vi "UI_Get_Application_Infos.vi"(8 "error in (no error)":errorcluster, 11 "Variant":variant) -> (0 "error out":errorcluster caption="sortie d'erreur", 3 "Variant Output":variant)   [LabVIEW 2018]
uses:
  controls/EXPERT_Inputs.ctl
  controls/DIGIT_5122_Inputs.ctl
  <instrlib>/niScope/Controls/niScope trigger source.ctl
  controls/HSDIO_6541_Inputs.ctl
  <instrlib>/niHSDIO/niHSDIO.llb/niHSDIO_ctl Trigger Source Values (Ring).ctl
  controls/SOFTWARE_Inputs.ctl
  controls/AO_6711_Inputs.ctl
  controls/AWG_5421_Inputs.ctl
  <instrlib>/niFgen/niFgen.llb/niFgen_ctl Trigger Source Values (Ring).ctl
  controls/XML_Inputs.ctl
  controls/EXPERT_Path_Selector.ctl
panel:
  in  "EXPERT Inputs":T1={"DIGIT 5122 Inputs"={"Sample Rate"=9.0, "Resource Name"="Digitizer", "Channel Name"="0", "Trigger Source"="VAL_EXTERNAL", "Vertical Range"=10.0, "Trigger Level"=3.0}, "HSDIO 6541 Inputs"={"Resource Name"="SequencerHSDIO", "Clock Rate"=1000000.0, "Trigger Source"="PFI0"}, "SOFTWARE Inputs"={"Application Directory"=path "D:/S.O.F.T.S/LABVIEW/PIL", "Software Version"="1.0.0", "Data Path"=path "D:/PIRENEA/DATA", "XML Path"=path "D:/PIRENEA/DATA", "XML File Filter"="*.xml", "XML Saved Path"=path "D:/PIRENEA/DATA", "Excit Scripts Path"=path "D:/PIRENEA/EXCIT_SCRIPTS", "Excit Scripts File Filter"="*.txt", "Excit Waveforms Path"=path "D:/PIRENEA/EXCIT_WFMS", "Excit Waveforms File Filter"="*.bin", "Timing Scripts Path"=path "D:/PIRENEA/SEQUENCE_SCRIPTS", "Timing Scripts File Filter"="*.txt", "Timing Waveforms Path"=path "D:/PIRENEA/SEQUENCE_WFMS", "Timing Waveforms File Filter"="*.bin", "Trapping Waveforms Path"=path "D:/PIRENEA/TRAPPING_WFMS", "Trapping Waveforms File Filter"="*.bin"}, "AO 6711 Inputs"={"Physical Channels"="AnalogOutput/ao0:3", "Min Voltage"=-10.0, "Max Voltage"=10.0, "Trigger Source"="/AnalogOutput/PFI0", "Counter"="AnalogOutput/ctr0"}, "AWG 5421 Inputs"={"Resource Name"="WaveformGenerator", "Sample Rate"=20000000.0, "Trigger Type"=2, "Trigger Source"="PFI0", "Waveform Gain"=0.31, "Digital Filter ON"=TRUE}, "XML Inputs"={"Version Tag Name"="XML_Version", "Version String"="1.0"}} {"AWG 5421 Inputs"."Sample Rate" format="%.2p"; "AWG 5421 Inputs"."Trigger Type" items=["None", "Software Edge", "Digital Edge", "Digital Level"]; "AO 6711 Inputs"."Max Voltage" min=-10.0 max=10.0; "AO 6711 Inputs"."Min Voltage" min=-10.0 max=10.0; "HSDIO 6541 Inputs"."Clock Rate" format="%.2p"; "DIGIT 5122 Inputs"."Trigger Level" format="%.2f"; "DIGIT 5122 Inputs"."Vertical Range" format="%.2f"; "DIGIT 5122 Inputs"."Sample Rate" step=65535.0 format="%#_3p"}
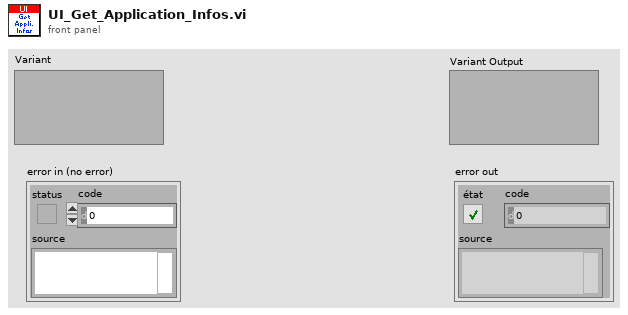
[diagram p1: front panel]
types:
  T1 = typedef "EXPERT_Inputs.ctl" = cluster{"DIGIT 5122 Inputs":T2, "HSDIO 6541 Inputs":T4, "SOFTWARE Inputs":T6, "AO 6711 Inputs":T7, "AWG 5421 Inputs":T8, "XML Inputs":T10}
  T2 = typedef "DIGIT_5122_Inputs.ctl" = cluster{"Sample Rate":dbl, "Resource Name":refnum<k15>, "Channel Name":string, "Trigger Source":T3, "Vertical Range":dbl, "Trigger Level":dbl}
  T3 = typedef "niScope trigger source.ctl" = string
  T4 = typedef "HSDIO_6541_Inputs.ctl" = cluster{"Resource Name":refnum<k15>, "Clock Rate":dbl, "Trigger Source":T5}
  T5 = typedef "niHSDIO_ctl Trigger Source Values (Ring).ctl" = string
  T6 = typedef "SOFTWARE_Inputs.ctl" = cluster{"Application Directory":path, "Software Version":string, "Data Path":path, "XML Path":path, "XML File Filter":string, "XML Saved Path":path, "Excit Scripts Path":path, "Excit Scripts File Filter":string, "Excit Waveforms Path":path, "Excit Waveforms File Filter":string, "Timing Scripts Path":path, "Timing Scripts File Filter":string, "Timing Waveforms Path":path, "Timing Waveforms File Filter":string, "Trapping Waveforms Path":path, "Trapping Waveforms File Filter":string}
  T7 = typedef "AO_6711_Inputs.ctl" = cluster{"Physical Channels":tag, "Min Voltage":dbl, "Max Voltage":dbl, "Trigger Source":tag, "Counter":tag}
  T8 = typedef "AWG_5421_Inputs.ctl" = cluster{"Resource Name":refnum<k15>, "Sample Rate":dbl, "Trigger Type":u16, "Trigger Source":T9, "Waveform Gain":dbl, "Digital Filter ON":bool}
  T9 = typedef "niFgen_ctl Trigger Source Values (Ring).ctl" = string
  T10 = typedef "XML_Inputs.ctl" = cluster{"Version Tag Name":string, "Version String":string}
  T11 = typedef "EXPERT_Path_Selector.ctl" = enum16{"Application", "Resources", "Data", "XML", "XML Saved", "Load Directory"}
  T12 = typedef "FileVersionInformation.ctl" = cluster{"FileVersion":string, "ProductName":string, "InternalName":string, "CompanyName":string, "LegalCopyright":string, "FileDescription":string}
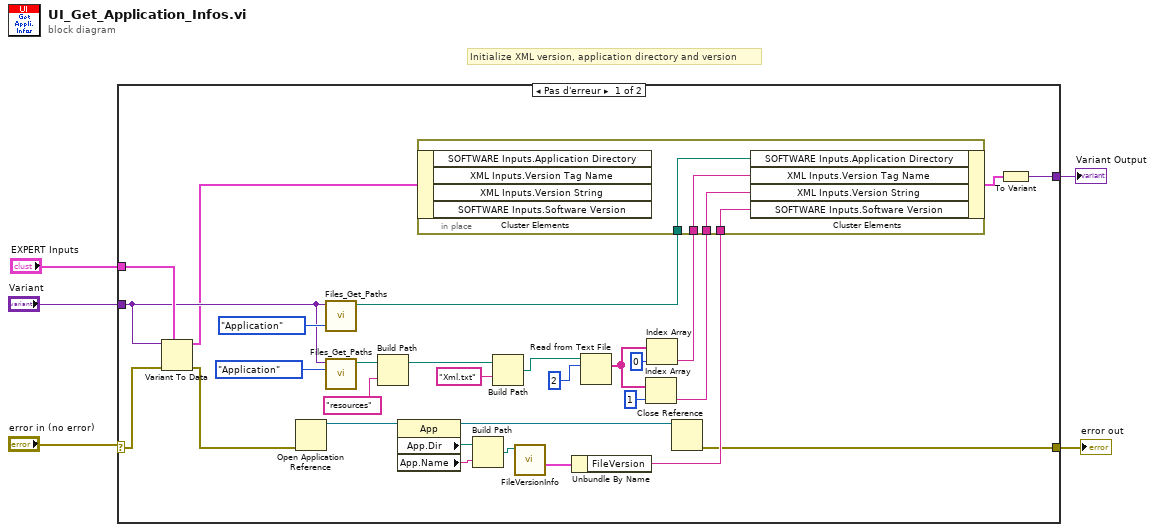
[diagram p0: block diagram]
diagram:
  # "Initialize XML version, application directory and version"
  n1 = case shown="Pas d'erreur" "error in (no error)" {
    selector: "error in (no error)" -> [w31 w40]
    tunnel: [w8 w40] -> w4
    tunnel: [w34 w39] -> w3
    tunnel: "Variant" -> [w21 w39]
    tunnel: "EXPERT Inputs" -> [w32 _]
    frame No Error {
      n2 = Variant To Data(error in=w31, type=w32, Variant=w21) -> (data=w20:T1, error out=w11:errorcluster)
      n3 = Open Application Reference(8:w11) -> (3:w12:refnum<vi>)  [unwired: 3 in, 1 out]
      n4 = call "Files_Get_Paths.vi"("EXPERT Path Selector"=EXPERT_Path_Selector."Application", "Variant"=w21) -> ("Path"=w19:path)  [unwired: 8 in, 1 out]
      n5 = call "Files_Get_Paths.vi"("EXPERT Path Selector"=EXPERT_Path_Selector."Application", "Variant"=w21) -> ("Path"=w23:path)  [unwired: 8 in, 1 out]
      n6 = Build Path(base path=w23, name or relative path="resources" ("nom ou chemin relatif")) -> (appended path=w7:path)
      n7 = property class="App"(reference=w12) -> (reference out=w9:refnum<vi>, "App.Dir"=w16:path, "App.Name"=w15:string)  [unwired: 1 in, 1 out]
      n8 = Build Path(base path=w16, name or relative path=w15) -> (appended path=w14:path)
      n9 = Build Path(base path=w7, name or relative path="Xml.txt" ("Version String")) -> (appended path=w28:path)
      n10 = call <vilib>:"FileVersionInfo.vi"("Application Path in"=w14) -> ("FileVersionInfo Out"=w13:T12)  [unwired: 7 in, 3 out]
      n11 = Unbundle By Name(w13) -> ("FileVersion"=w10:string)
      n12 = Read from Text File(file (use dialog)=w28, count=2 ("nombre")) -> (text=w26:string[])  [unwired: 2 in, 3 out]
      n13 = Index Array(array=w26, index=1 ("indice")) -> (element=w17:string)
      n14 = Index Array(array=w26, index=0 ("indice")) -> (element=w18:string)
      n15 = in-place {
        in-place-border: w19 -> [w38]
        in-place-border: w18 -> [w36]
        in-place-border: w17 -> [w37]
        in-place-border: w10 -> [w35]
        n16 = in-place-cluster #1(w20) -> ()  [unwired: 4 out]
        n17 = in-place-cluster #1("SOFTWARE Inputs.Application Directory"=w38, "XML Inputs.Version Tag Name"=w36, "XML Inputs.Version String"=w37, "SOFTWARE Inputs.Software Version"=w35) -> (w33:T1)
      }
      n18 = Close Reference(reference=w9) -> (error out=w8:errorcluster)  [unwired: 1 in]
      n19 = To Variant(anything=w33) -> (Variant=w34:variant)
    }
    frame Error {
    }
  }
  "error out" <- w4
  "Variant Output" <- w3
